vi "Display SLM.vi"(2 "Action":u16(ring) items=["Read", "Initialize"], 7 "displayed matrix":u8[][](array[numeric])=array600x792[475200 elements]) -> (13 "Read action":u16)   [LabVIEW 2014]
panel:
  in  "number":dbl=3840.0
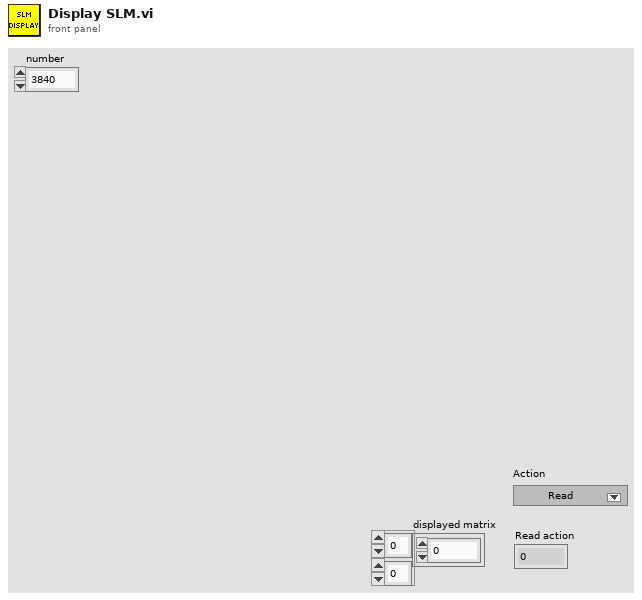
[diagram p1: front panel]
types:
  T1 = typedef "IMAQ Image.ctl" = refnum<image>
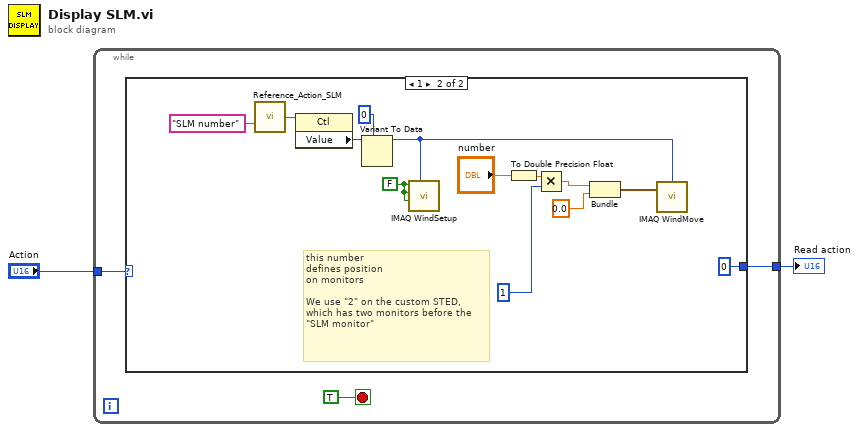
[diagram p0: block diagram]
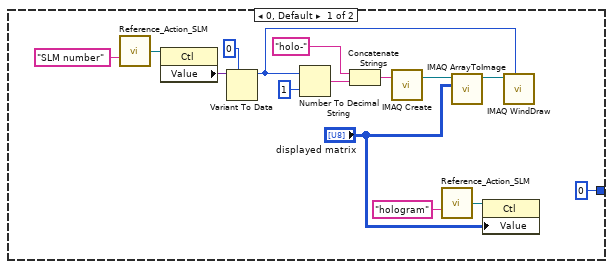
[diagram p2: hidden frame]
diagram:
  n1 = while {
    tunnel: "Action" -> [w4]
    tunnel: [w3] -> w1
    stop <- TRUE stop-if-true
    n2 = case shown="1" w4 {
      tunnel: [u16 0 ("Action 2") u16 0 ("Action 2")] -> w3
      frame 0, Default {
        n3 = call "Reference_Action_SLM.vi"("Control Name"="SLM number") -> ("Ref OUT"=w15:refnum<vi>)  [unwired: 12 in, 2 out]
        n4 = property class="Ctl"(reference=w15) -> ("Value"=w16:variant)  [unwired: 1 in, 2 out]
        n5 = Variant To Data(type=0, Variant=w16) -> (data=w10:i32)  [unwired: 1 in, 1 out]
        n6 = Number To Decimal String(number=w10, width (-)=i16 1) -> (decimal integer string=w19:string)
        n7 = Concatenate Strings("holo-", w19) -> (w12:string)
        n8 = call "IMAQ Create"("Image Name"=w12) -> ("New Image"=w11:T1)  [unwired: 3 in, 2 out]
        n9 = call "Reference_Action_SLM.vi"("Control Name"="hologram") -> ("Ref OUT"=w8:refnum<vi>)  [unwired: 12 in, 2 out]
        n10 = call "IMAQ ArrayToImage"("Image Pixels (U8)"="displayed matrix", "Image"=w11) -> ("Image Out"=w20:T1)  [unwired: 4 in, 5 out]
        n11 = property class="Ctl"(reference=w8, "Value"="displayed matrix") -> ()  [unwired: 1 in, 2 out]
        n12 = call "IMAQ WindDraw"("Window Number (0...15)"=w10, "Image"=w20) -> ()  [unwired: 4 in, 6 out]
      }
      frame 1 {
        w33 = FALSE ("Window can grow? (Yes)")
        # "this number\ndefines position\non monitors\n\nWe use \"2\" on the custom STED, which has two monitors before the \"SLM monitor\""
        n13 = call "Reference_Action_SLM.vi"("Control Name"="SLM number") -> ("Ref OUT"=w30:refnum<vi>)  [unwired: 12 in, 2 out]
        n14 = property class="Ctl"(reference=w30) -> ("Value"=w31:variant)  [unwired: 1 in, 2 out]
        n15 = Variant To Data(type=0, Variant=w31) -> (data=w28:i32)  [unwired: 1 in, 1 out]
        n16 = call "IMAQ WindSetup"("Window Number (0...15)"=w28, "Window has title bar? (Yes)"=w33, "Window can close? (Yes)"=w33, "Window can grow? (Yes)"=w33) -> ()  [unwired: 3 in, 5 out]
        n17 = To Double Precision Float(number="number") -> (double precision float=w23:dbl)
        n18 = Multiply(x=w23, y=1) -> (x*y=w25:dbl)
        n19 = Bundle(w25, 0.0) -> (w26:cluster{dbl, dbl})  [unwired: 1 out]
        n20 = call "IMAQ WindMove"("Window Number (0...15)"=w28, "Coordinates (screen)"=w26) -> ()  [unwired: 2 in, 3 out]
      }
    }
  }
  "Read action" <- w1
